vi "Calculate_bottle_distance_matrix.vi"(2 "Odour component data":T2={"names"=["Benzaldehyde", "Benzene", "Butyraldehyde", "Butyric acid", "Formic acid", "Coumarin", "Ocanal", "Guaiacol", "Octanol", "Propionate", "Vanillin", "Cineole", "Eugenol ", "Methyl salicylate", "Phenylethanol", "Pentanol", "Dichloromethane", "Methyl butanol", "Dimethylacetophenone", "Ethylphenol", "Methylnaphthalene", "Dimethoxybenzene", "Methoxy methylphenol", "Phenylpropionaldehyde", "Methyl benzoate", "Acetophenone", "S-Carvone", "gamma-Terpinene", "alpha-Terpinene", "Tripropylamine", "Ethyl butyrate", "Ethyl heptanoate", "Isopentylamine", "Ethyl isovalerate", "Cyclohexanol", "Valeric acid", "Propyl acetate", "Ethyl formate", "Heptanone", "Valeraldehyde", "Heptanoic acid ", "Hexanol", "Nonanoic acid", "Decanol", "Undecanal", "Lauric aldehyde", "Methylacetophenone", "Methyl anthranilate", "Ethylhexanoic acid", "Benzyl acetate", "Allylanisole", "Citronellol", "Ethyl acetate", "Hexanoic acid", "Nonanol", "Allylbenzene", "Citronellic acid", "Ethyl valerate", "Isobutyl proprionate", "Methyl butyrate", "Methyl valerate", "Pentyl acetate", "Nonanone", "Methylheptanoic acid", "Fenchone", "Octadecylamine", "Phenyl butanone", "S-Limonene", "Menthone", "Phenyl acetate", "Ethyl caproate", "Nonanal", "Methyloctanoic acid", "Methylanisol", "Sesamol", "Cinnamaldehyde", "Anethole", "Geraniol", "Geranyl acetate", "Ethyl tiglate", "Hexenyl tiglate", "Hydroxacetophenone"], "CID"=[240, 241, 261, 264, 284, 323, 454, 460, 957, 1032, 1183, 2758, 3314, 4133, 6054, 6276, 6344, 6405, 6985, 6997, 7002, 7043, 7144, 7146, 7150, 7410, 7439, 7461, 7462, 7616, 7762, 7797, 7894, 7945, 7966, 7991, 7997, 8025, 8051, 8063, 8094, 8103, 8158, 8174, 8186, 8194, 8500, 8635, 8697, 8785, 8815, 8842, 8857, 8892, 8914, 9309, 10402, 10882, 10895, 12180, 12206, 12348, 13187, 14475, 14525, 15793, 17355, 22311, 26447, 31229, 31265, 31289, 62089, 66353, 68289, 637511, 637563, 637566, 1549026, 5281163, 15461361, 24868161], "volatility"=[1.27, 94.8, 111.0, 1.65, 42.59, 0.00098, 1.18, 0.103, 0.0794, 3.53, 0.000118, 1.9, 0.0221, 0.0343, 0.09, 2.2, 435.0, 16.7, 0.063, 0.153, 0.067, 0.47, 0.078, 0.27, 0.38, 0.45, 0.115, 1.09, 1.6, 1.51, 11.3, 0.68, 51.1, 8.3, 0.657, 0.196, 35.9, 244.62, 3.85, 26.0, 0.0107, 0.928, 0.00165, 0.00851, 0.083, 0.02, 0.159, 0.0271, 0.03, 0.177, 0.165, 0.02, 93.2, 0.0435, 0.0227, 3.6, 0.005, 4.8, 6.47, 32.3, 19.15, 3.5, 1.6, 0.018, 0.82, 4.4e-05, 0.1, 1.64, 0.28, 0.4, 1.665, 0.37, 0.006, 1.9, 0.00689, 0.03, 0.07, 0.03, 0.03, 4.269, 0.0306, 0.0856], "2D map"=[[-35.65469956598489, 270.2139888611614], [98.13934241781413, 398.7044129905194], [233.76965217524653, 190.396254515234], [150.23211981471368, 221.1580180551867], [297.4652966197888, 315.17787277483853], [-231.36430031040578, 203.83961706757722], [207.17154717294608, -174.93797693620664], [-152.674775911407, 243.13326408951488], [251.79971870928094, -161.91563269564605], [185.8537823396016, 288.33901581648973], [-262.41250467128555, 75.06909387065261], [179.59046460245207, -56.04022976112759], [-317.9647981045101, -43.831335920252606], [-294.6567457719659, 122.4114919562466], [-126.91499848915312, 102.91867516437394], [281.28159545024744, 102.71121558509061], [339.8533239503384, 251.5898534107341], [204.32713615045907, 160.28624069412643], [-273.35122450752266, -42.263086129371295], [-111.19908951088753, 208.56819115230442], [-294.76791641311274, 191.0620800004279], [-191.8219737813257, 189.9450263215761], [-191.41524828002733, 142.3631394442883], [-159.5151592759888, 8.436616623045376], [-232.541000525234, 130.6588221918013], [-122.94463556800827, 191.9015477463772], [-208.04948323720893, -158.23331010430897], [-244.97562606669857, -207.08642326769737], [-246.95298712232488, -204.5270138088883], [256.9928159423369, -68.61957940549138], [14.89385579391006, 133.32677712624545], [51.353048668431704, -178.40967800200966], [258.01381231117176, 146.47302969001294], [-2.8949993967070853, 37.62756232510908], [180.22600495656366, 104.35598527492789], [110.87943807753645, 170.98018005743705], [51.170561159934444, 191.40195381349582], [147.75453833538387, 281.1287978570423], [119.41963149938562, -28.685096728203234], [236.49773623152166, 93.65722557836662], [114.59724760685786, -96.63812347643292], [266.82605746771884, 13.479384089782926], [114.07056457899871, -243.76771476212969], [252.76854811630145, -250.34883594312083], [205.2249479165084, -308.24507263086724], [213.71781772180816, -327.1617713637844], [-235.0545852465996, -26.650521263465556], [-296.4544615523987, 107.12891384196561], [-26.698853099282278, -87.93548942481429], [-165.64242245257407, -73.95049456240373], [-236.20336645538308, -104.36500693122969], [10.245213827208765, -277.3638544350568], [93.81548252939837, 259.6981542624837], [112.29360419618213, 39.85287306331019], [249.27752347690375, -213.31743810727397], [-120.17144764398293, 295.9933132570569], [-29.645616081049297, -281.62183144789145], [17.20580648407221, -8.697992950423888], [-19.733594212360888, 18.78620227069331], [37.27700380001177, 217.8007894783545], [31.18693554024182, 86.77073317156534], [47.27018090750722, -66.65120683967478], [143.47309690220376, -211.27776405264314], [12.179301078164926, -164.80443024342875], [-158.52742292807153, -249.66981496564088], [396.3821953927539, -294.1625463085245], [-152.14035558594634, -143.60083658864872], [-252.7110045881726, -217.6654971930947], [-148.46677914865614, -213.0788157505672], [-187.82662250571298, 101.29743735356698], [21.156685543603103, -115.32895882976128], [197.2464957982167, -238.619079383165], [58.40307821935197, -228.79990905087422], [-210.9178904519634, 38.88407874545689], [-213.3415540440491, 296.65536658552134], [-303.9529163482059, 9.54512145075226], [-269.340230018179, -95.83774156123017], [-23.502678410472118, -253.81154308548392], [-79.59753085274536, -324.2771585204367], [-58.24361669961045, 130.29205926060382], [-76.44304440140283, -273.6441237325548], [515.3849497534994, -68.17744072149127]], "distance matrix"=array82x82[6724 elements]}, 3 "Odour bottles":T1(array[cluster])) -> (0 "Colour grid":u32[][](array[numeric]))   [LabVIEW 2016]
panel:
  out "Similarities":dbl[][](array[numeric])
  out "DistanceMatrixColorBox":u32[][](array[colorbox])=[[16777215, 16777215, 16777215, 16777215, 16777215, 16777215, 16777215, 16777215, 16777215, 16777215, 16777215, 16777215, 16777215, 16777215, 16777215, 16777215], [16777215, 16777215, 16777215, 16777215, 16777215, 16777215, 16777215, 16777215, 16777215, 16777215, 16777215, 16777215, 16777215, 16777215, 16777215, 16777215], [16777215, 16777215, 16777215, 16777215, 16777215, 16777215, 16777215, 16777215, 16777215, 16777215, 16777215, 16777215, 16777215, 16777215, 16777215, 16777215], [16777215, 16777215, 16777215, 16777215, 16777215, 16777215, 16777215, 16777215, 16777215, 16777215, 16777215, 16777215, 16777215, 16777215, 16777215, 16777215], [16777215, 16777215, 16777215, 16777215, 16777215, 16777215, 16777215, 16777215, 16777215, 16777215, 16777215, 16777215, 16777215, 16777215, 16777215, 16777215], [16777215, 16777215, 16777215, 16777215, 16777215, 16777215, 16777215, 16777215, 16777215, 16777215, 16777215, 16777215, 16777215, 16777215, 16777215, 16777215], [16777215, 16777215, 16777215, 16777215, 16777215, 16777215, 16777215, 16777215, 16777215, 16777215, 16777215, 16777215, 16777215, 16777215, 16777215, 16777215], [16777215, 16777215, 16777215, 16777215, 16777215, 16777215, 16777215, 16777215, 16777215, 16777215, 16777215, 16777215, 16777215, 16777215, 16777215, 16777215], [16777215, 16777215, 16777215, 16777215, 16777215, 16777215, 16777215, 16777215, 16777215, 16777215, 16777215, 16777215, 16777215, 16777215, 16777215, 16777215], [16777215, 16777215, 16777215, 16777215, 16777215, 16777215, 16777215, 16777215, 16777215, 16777215, 16777215, 16777215, 16777215, 16777215, 16777215, 16777215], [16777215, 16777215, 16777215, 16777215, 16777215, 16777215, 16777215, 16777215, 16777215, 16777215, 16777215, 16777215, 16777215, 16777215, 16777215, 16777215], [16777215, 16777215, 16777215, 16777215, 16777215, 16777215, 16777215, 16777215, 16777215, 16777215, 16777215, 16777215, 16777215, 16777215, 16777215, 16777215], [16777215, 16777215, 16777215, 16777215, 16777215, 16777215, 16777215, 16777215, 16777215, 16777215, 16777215, 16777215, 16777215, 16777215, 16777215, 16777215], [16777215, 16777215, 16777215, 16777215, 16777215, 16777215, 16777215, 16777215, 16777215, 16777215, 16777215, 16777215, 16777215, 16777215, 16777215, 16777215], [16777215, 16777215, 16777215, 16777215, 16777215, 16777215, 16777215, 16777215, 16777215, 16777215, 16777215, 16777215, 16777215, 16777215, 16777215, 16777215], [16777215, 16777215, 16777215, 16777215, 16777215, 16777215, 16777215, 16777215, 16777215, 16777215, 16777215, 16777215, 16777215, 16777215, 16777215, 16777215]]
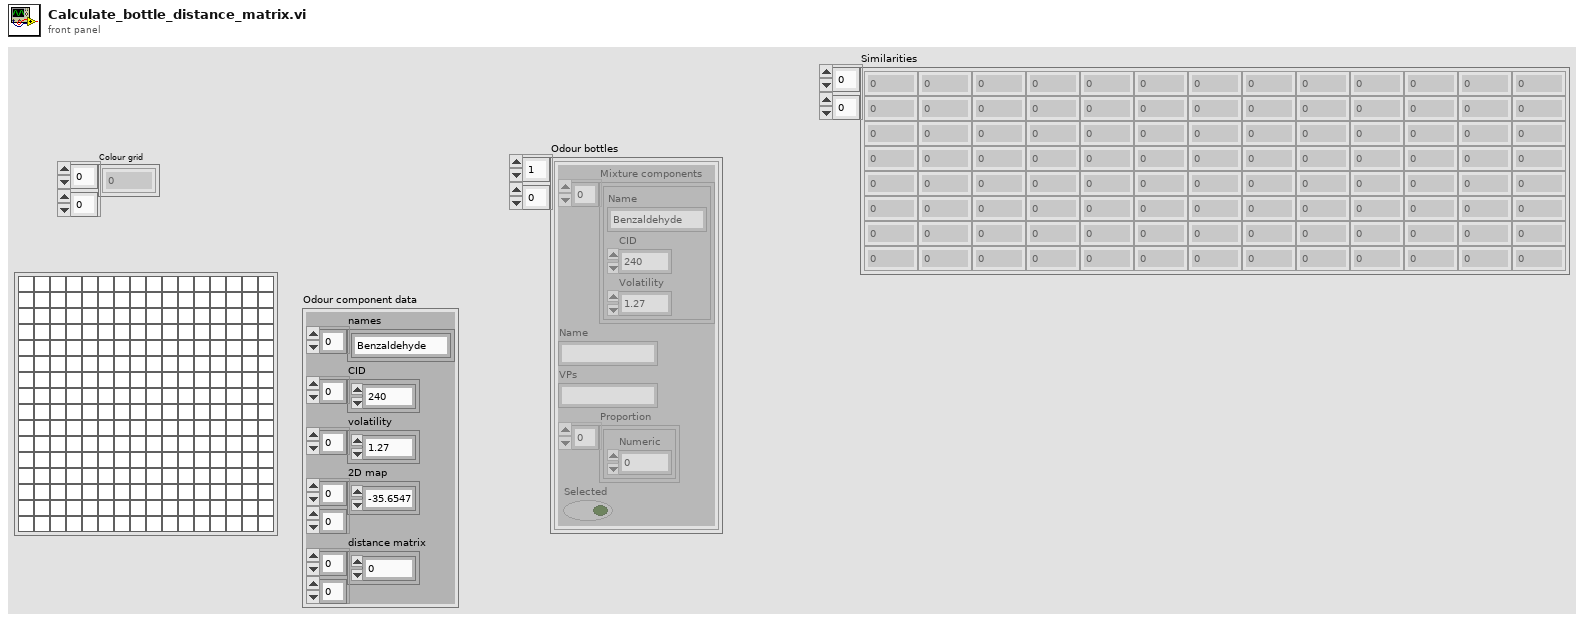
[diagram p1: front panel]
types:
  T1 = cluster{"Mixture components":cluster{"Name":string, "CID":i32, "Volatility":dbl}[], "Name":string, "VPs":string, "Proportion":cluster{"Numeric":dbl}[], "Selected":bool}[][]
  T2 = cluster{"names":string[], "CID":i32[], "volatility":dbl[], "2D map":dbl[][], "distance matrix":dbl[][]}
  T3 = cluster{"Mixture components":cluster{"Name":string, "CID":i32, "Volatility":dbl}[], "Name":string, "VPs":string, "Proportion":cluster{"Numeric":dbl}[], "Selected":bool}[]
  T4 = cluster{"Name":string, "CID":i32, "Volatility":dbl}[]
  T5 = cluster{"Name":string, "CID":i32, "Volatility":dbl}
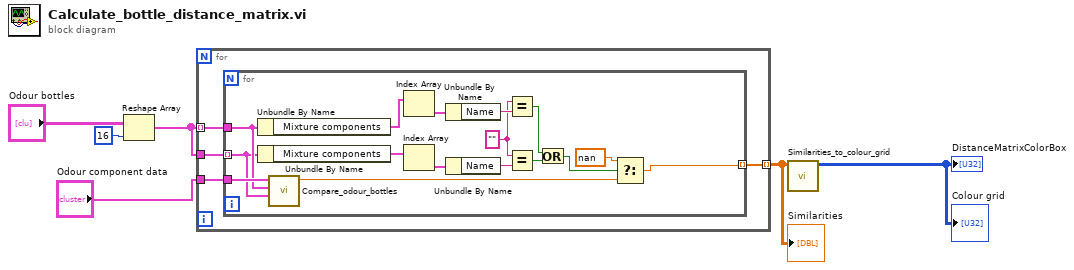
[diagram p0: block diagram]
diagram:
  n1 = Reshape Array("Odour bottles", 16 ("dimension size")) -> (w2:T3)
  n2 = for {
    tunnel: w2 -> [w10] mode=indexing
    tunnel: w2 -> [w9]
    tunnel: [w8] -> w4 mode=indexing
    tunnel: "Odour component data" -> [w7]
    n3 = for {
      tunnel: w10 -> [w25]
      tunnel: w9 -> [w20] mode=indexing
      tunnel: [w11] -> w8 mode=indexing
      tunnel: w7 -> [w26]
      w17 = "" ("x")
      n4 = Unbundle By Name(w25) -> ("Mixture components"=w24:T4)
      n5 = Unbundle By Name(w20) -> ("Mixture components"=w21:T4)
      n6 = call "Compare_odour_bottles.vi"("Bottle 2"=w20, "Bottle 1"=w25, "Odour component data"=w26) -> ("distance"=w12:dbl)  [unwired: 8 in]
      n7 = Index Array(array=w24) -> (element=w23:T5)  [unwired: 1 in]
      n8 = Index Array(array=w21) -> (element=w22:T5)  [unwired: 1 in]
      n9 = Unbundle By Name(w23) -> ("Name"=w19:string)
      n10 = Unbundle By Name(w22) -> ("Name"=w16:string)
      n11 = Equal?(x=w17, y=w19) -> (x = y?=w18:bool)
      n12 = Equal?(x=w17, y=w16) -> (x = y?=w15:bool)
      n13 = Or(x=w18, y=w15) -> (x .or. y?=w14:bool)
      n14 = Select(t=nan, s=w14, f=w12) -> (s? t:f=w11:dbl)
    }
  }
  "Similarities" <- w4
  n15 = call "Similarities_to_colour_grid.vi"("Array in"=w4) -> ("Array out"=→"Colour grid" →"DistanceMatrixColorBox":u32[][])  [unwired: 10 in]
